vi "transfer table data.vi"(9 "transfer specification in":T1[](array[typedef]), 10 "data table source in":T3, 11 "data table sink in":T3) -> (1 "transfer specification out":T1[](array[typedef]), 2 "data table source out":T3, 3 "data table sink out":T3)   [LabVIEW 2013, in "tag bus.lvlib" / "data table.lvlib"]
doc: "Applies the data transfer between the source table and sink table, as defined by the transfer specification."
uses:
  data table.lvlib
  data table.ctl
  transfer specification.ctl
  tag/Data Type.ctl
  tag/tag descriptor.lvclass
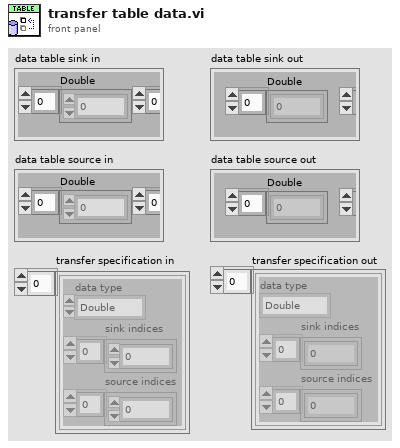
[diagram p1: front panel]
types:
  T1 = typedef "tag bus.lvlib/data table.lvlib/transfer specification.ctl" = cluster{"data type":T2, "sink indices":i32[], "source indices":i32[]}
  T2 = typedef "tag bus.lvlib/tag descriptor.lvclass/Data Type.ctl" = enum16{"Double", "Single", "I64", "I32", "I16", "I8", "U64", "U32", "U16", "U8", "Boolean", "String", "Array of Double", "Array of Single", "Array of I64", "Array of I32", "Array of I16", "Array of I8", "Array of U64", "Array of U32", "Array of U16", "Array of U8", "Array of Boolean", "Array of String"}
  T3 = typedef "tag bus.lvlib/data table.lvlib/data table.ctl" = cluster{"Double":dbl[], "Single":sgl[], "I64":i64[], "I32":i32[], "I16":i16[], "I8":i8[], "U64":u64[], "U32":u32[], "U16":u16[], "U8":u8[], "Boolean":bool[], "String":string[], "Array of Double":cluster{"DBL Array":dbl[]}[], "Array of Single":cluster{"SGL Array":sgl[]}[], "Array of I64":cluster{"I64 Array":i64[]}[], "Array of I32":cluster{"I32 Array":i32[]}[], "Array of I16":cluster{"I16 Array":i16[]}[], "Array of I8":cluster{"I8 Array":i8[]}[], "Array of U64":cluster{"U64 Array":u64[]}[], "Array of U32":cluster{"U32 Array":u32[]}[], "Array of U16":cluster{"U16 Array":u16[]}[], "Array of U8":cluster{"U8 Array":u8[]}[], "Array of Boolean":cluster{"Boolean Array":bool[]}[], "Array of String":cluster{"String Array":string[]}[]}
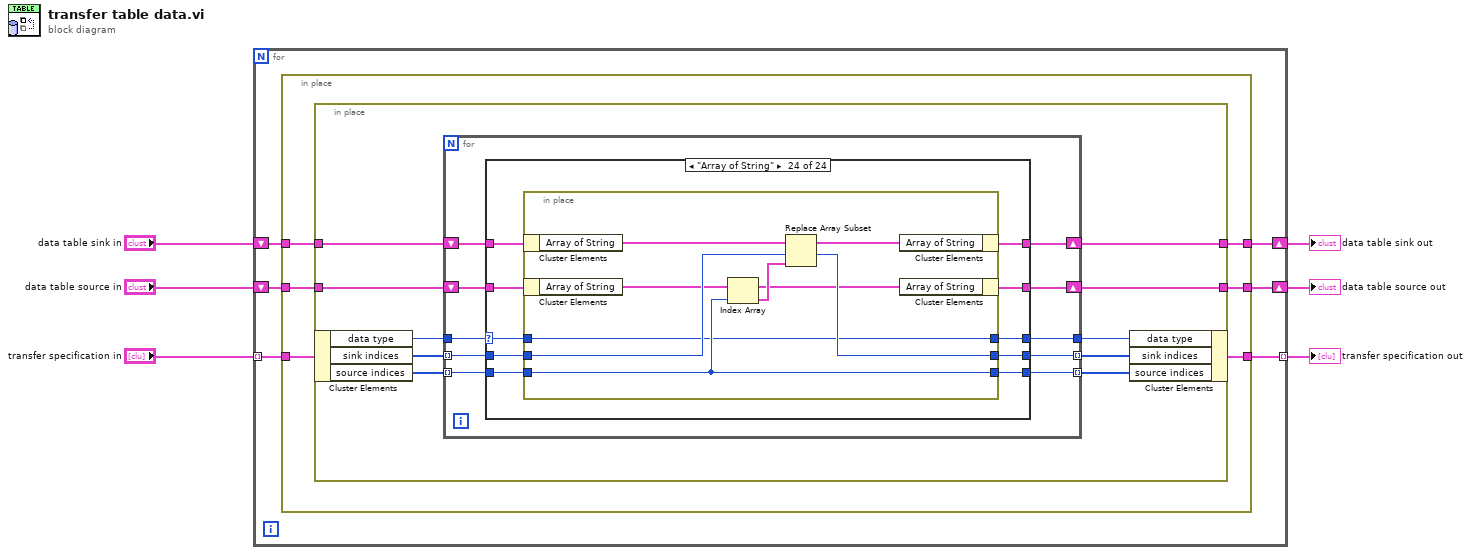
[diagram p0: block diagram]
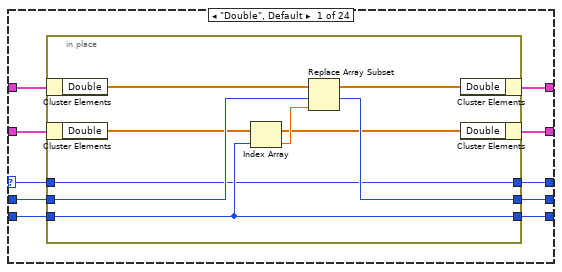
[diagram p2: hidden frame]
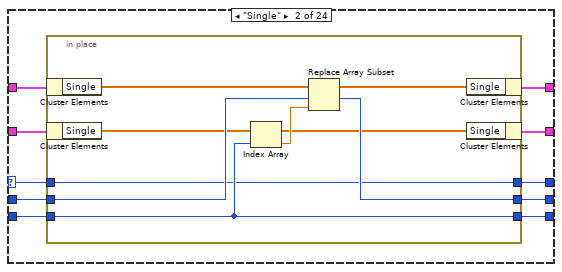
[diagram p3: hidden frame]
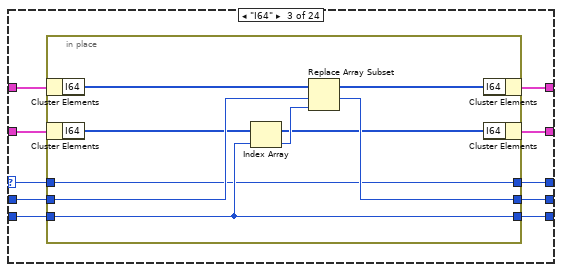
[diagram p4: hidden frame]
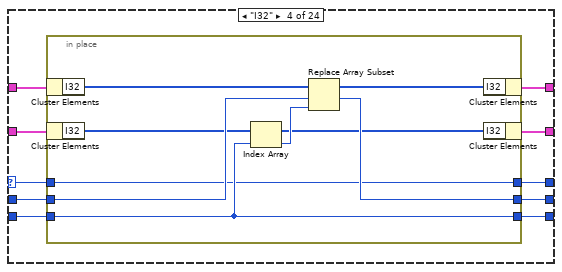
[diagram p5: hidden frame]
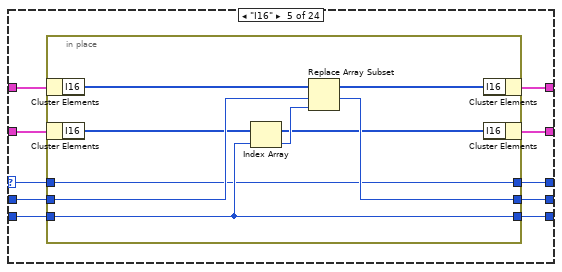
[diagram p6: hidden frame]
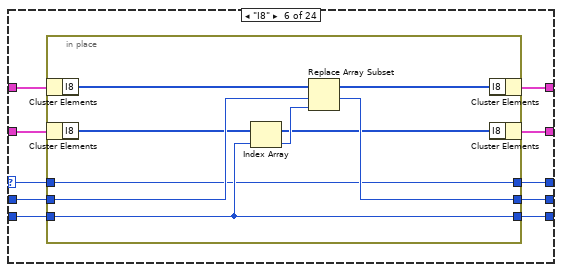
[diagram p7: hidden frame]
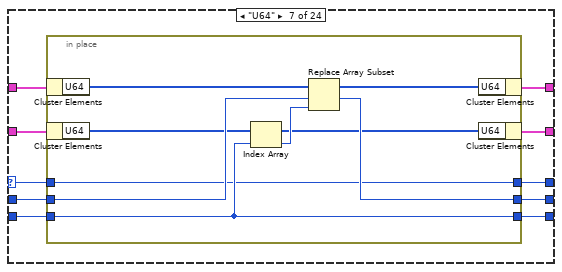
[diagram p8: hidden frame]
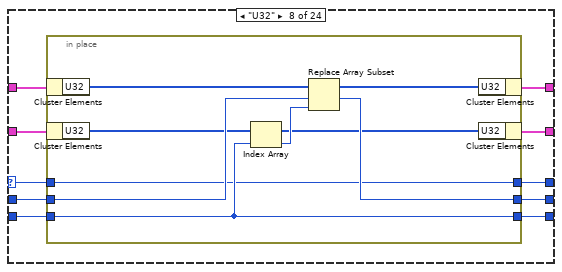
[diagram p9: hidden frame]
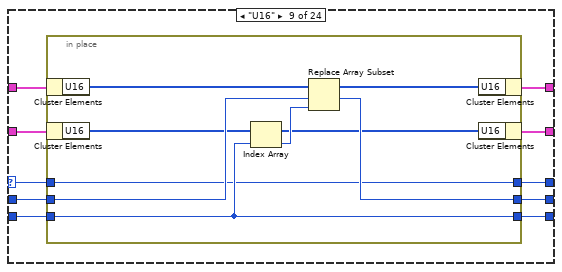
[diagram p10: hidden frame]
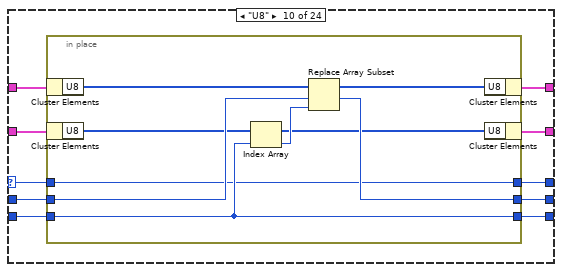
[diagram p11: hidden frame]
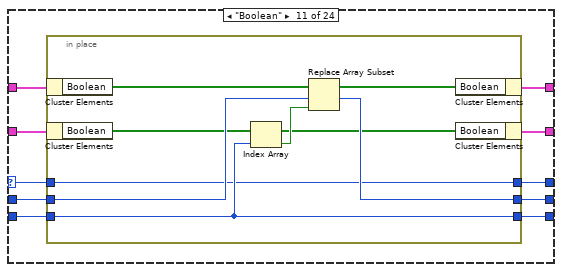
[diagram p12: hidden frame]
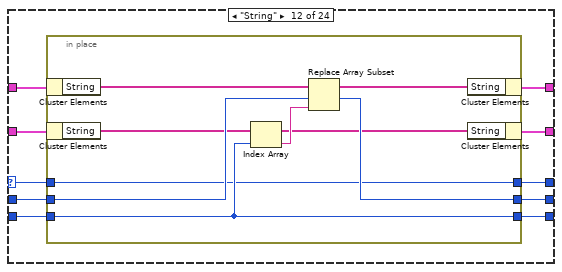
[diagram p13: hidden frame]
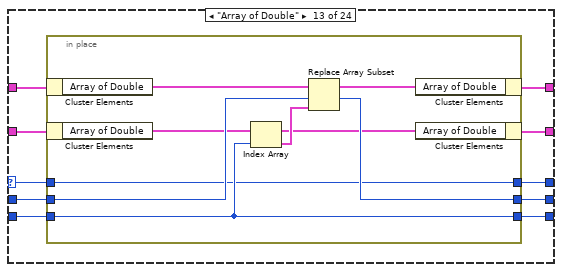
[diagram p14: hidden frame]
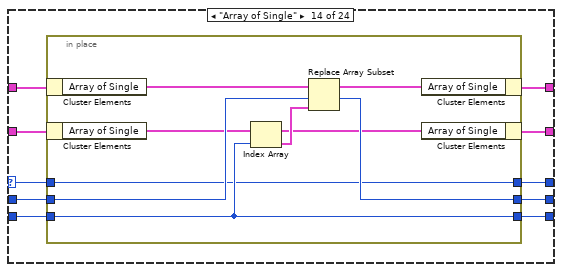
[diagram p15: hidden frame]
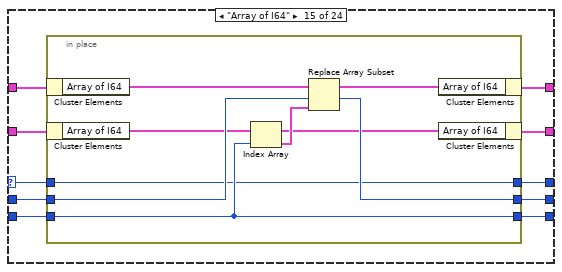
[diagram p16: hidden frame]
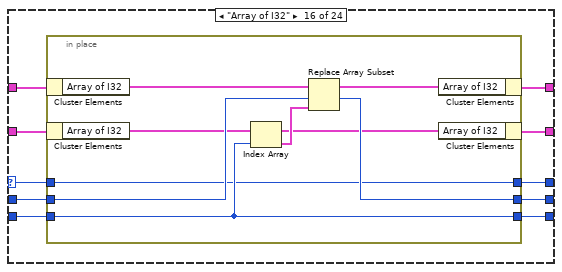
[diagram p17: hidden frame]
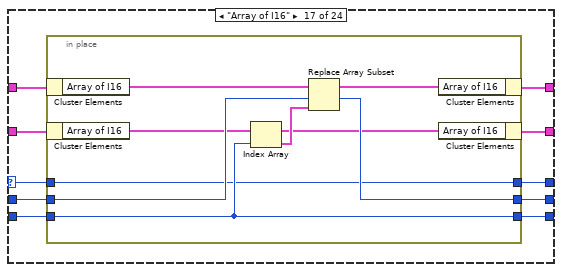
[diagram p18: hidden frame]
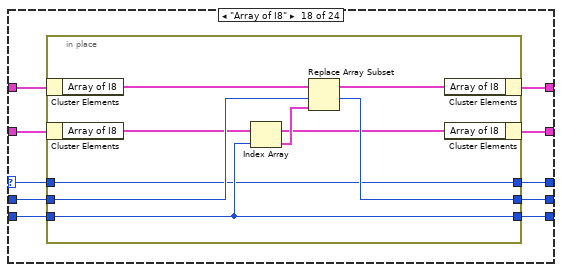
[diagram p19: hidden frame]
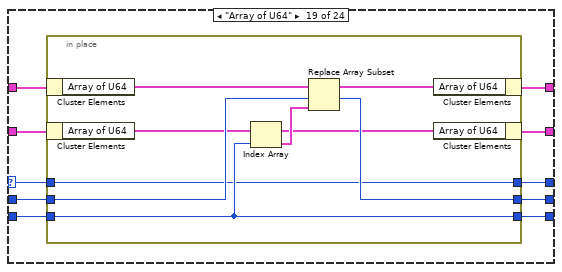
[diagram p20: hidden frame]
diagram:
  n1 = for {
    tunnel: "transfer specification in" -> [w8] mode=indexing
    shift-right: [w9] -> w2
    shift-left: "data table source in" -> [w10]
    shift-right: [w11] -> w3
    shift-left: "data table sink in" -> [w12]
    tunnel: [w7] -> w1 mode=indexing
    n2 = in-place {
      in-place-border: w12 -> [w18]
      in-place-border: [w17] -> w11
      in-place-border: w10 -> [w16]
      in-place-border: [w15] -> w9
      in-place-border: w8 -> [w14]
      in-place-border: [w13] -> w7
      n3 = in-place {
        in-place-border: w18 -> [w28]
        in-place-border: [w27] -> w17
        in-place-border: w16 -> [w26]
        in-place-border: [w25] -> w15
        n4 = in-place-cluster #1(w14) -> ("data type"=w24:T2, "sink indices"=w23:i32[], "source indices"=w22:i32[])
        n5 = for {
          shift-right: [w36] -> w27
          shift-left: w28 -> [w37]
          shift-right: [w35] -> w25
          shift-left: w26 -> [w34]
          tunnel: w24 -> [w38]
          tunnel: w23 -> [w33] mode=indexing
          tunnel: w22 -> [w32] mode=indexing
          tunnel: [w31] -> w21 mode=indexing
          tunnel: [w30] -> w20 mode=indexing
          tunnel: [w29] -> w19
          n6 = case shown="\"Array of String\"" w38 {
            selector: w38 -> [w40 w57 w74 w91 w108 w125 w142 w159 w176 w193 w210 w227 w244 w261 w278 w295 w312 w329 w346 w363 w380 w397 w414 w431]
            tunnel: w37 -> [w48 w65 w82 w99 w116 w133 w150 w167 w184 w201 w218 w235 w252 w269 w286 w303 w320 w337 w354 w371 w388 w405 w422 w439]
            tunnel: [w46 w63 w80 w97 w114 w131 w148 w165 w182 w199 w216 w233 w250 w267 w284 w301 w318 w335 w352 w369 w386 w403 w420 w437] -> w36
            tunnel: [w45 w62 w79 w96 w113 w130 w147 w164 w181 w198 w215 w232 w249 w266 w283 w300 w317 w334 w351 w368 w385 w402 w419 w436] -> w35
            tunnel: w34 -> [w47 w64 w81 w98 w115 w132 w149 w166 w183 w200 w217 w234 w251 w268 w285 w302 w319 w336 w353 w370 w387 w404 w421 w438]
            tunnel: w33 -> [w44 w61 w78 w95 w112 w129 w146 w163 w180 w197 w214 w231 w248 w265 w282 w299 w316 w333 w350 w367 w384 w401 w418 w435]
            tunnel: w32 -> [w43 w60 w77 w94 w111 w128 w145 w162 w179 w196 w213 w230 w247 w264 w281 w298 w315 w332 w349 w366 w383 w400 w417 w434]
            tunnel: [w42 w59 w76 w93 w110 w127 w144 w161 w178 w195 w212 w229 w246 w263 w280 w297 w314 w331 w348 w365 w382 w399 w416 w433] -> w31
            tunnel: [w41 w58 w75 w92 w109 w126 w143 w160 w177 w194 w211 w228 w245 w262 w279 w296 w313 w330 w347 w364 w381 w398 w415 w432] -> w30
            tunnel: [w39 w56 w73 w90 w107 w124 w141 w158 w175 w192 w209 w226 w243 w260 w277 w294 w311 w328 w345 w362 w379 w396 w413 w430] -> w29
            frame "Double", Default {
              n7 = in-place {
                in-place-border: w44 -> [w53]
                in-place-border: w43 -> [w52]
                in-place-border: [w53] -> w42
                in-place-border: [w52] -> w41
                in-place-border: w40 -> [w51]
                in-place-border: [w51] -> w39
                n8 = in-place-cluster #2(w48) -> ("Double"=w55:dbl[])
                n9 = in-place-cluster #3(w47) -> ("Double"=w49:dbl[])
                n10 = Index Array(array=w49, index=w52) -> (element=w50:dbl)
                n11 = Replace Array Subset(array=w55, new element=w50, index=w53) -> (w54:dbl[])
                n12 = in-place-cluster #2("Double"=w54) -> (w46:T3)
                n13 = in-place-cluster #3("Double"=w49) -> (w45:T3)
              }
            }
            frame "Single" {
              n14 = in-place {
                in-place-border: w61 -> [w70]
                in-place-border: w60 -> [w69]
                in-place-border: [w70] -> w59
                in-place-border: [w69] -> w58
                in-place-border: w57 -> [w68]
                in-place-border: [w68] -> w56
                n15 = in-place-cluster #4(w65) -> ("Single"=w72:sgl[])
                n16 = in-place-cluster #5(w64) -> ("Single"=w66:sgl[])
                n17 = Index Array(array=w66, index=w69) -> (element=w67:sgl)
                n18 = Replace Array Subset(array=w72, new element=w67, index=w70) -> (w71:sgl[])
                n19 = in-place-cluster #4("Single"=w71) -> (w63:T3)
                n20 = in-place-cluster #5("Single"=w66) -> (w62:T3)
              }
            }
            frame "I64" {
              n21 = in-place {
                in-place-border: w78 -> [w87]
                in-place-border: w77 -> [w86]
                in-place-border: [w87] -> w76
                in-place-border: [w86] -> w75
                in-place-border: w74 -> [w85]
                in-place-border: [w85] -> w73
                n22 = in-place-cluster #6(w82) -> ("I64"=w89:i64[])
                n23 = in-place-cluster #7(w81) -> ("I64"=w83:i64[])
                n24 = Index Array(array=w83, index=w86) -> (element=w84:i64)
                n25 = Replace Array Subset(array=w89, new element=w84, index=w87) -> (w88:i64[])
                n26 = in-place-cluster #6("I64"=w88) -> (w80:T3)
                n27 = in-place-cluster #7("I64"=w83) -> (w79:T3)
              }
            }
            frame "I32" {
              n28 = in-place {
                in-place-border: w95 -> [w104]
                in-place-border: w94 -> [w103]
                in-place-border: [w104] -> w93
                in-place-border: [w103] -> w92
                in-place-border: w91 -> [w102]
                in-place-border: [w102] -> w90
                n29 = in-place-cluster #8(w99) -> ("I32"=w106:i32[])
                n30 = in-place-cluster #9(w98) -> ("I32"=w100:i32[])
                n31 = Index Array(array=w100, index=w103) -> (element=w101:i32)
                n32 = Replace Array Subset(array=w106, new element=w101, index=w104) -> (w105:i32[])
                n33 = in-place-cluster #8("I32"=w105) -> (w97:T3)
                n34 = in-place-cluster #9("I32"=w100) -> (w96:T3)
              }
            }
            frame "I16" {
              n35 = in-place {
                in-place-border: w112 -> [w121]
                in-place-border: w111 -> [w120]
                in-place-border: [w121] -> w110
                in-place-border: [w120] -> w109
                in-place-border: w108 -> [w119]
                in-place-border: [w119] -> w107
                n36 = in-place-cluster #10(w116) -> ("I16"=w123:i16[])
                n37 = in-place-cluster #11(w115) -> ("I16"=w117:i16[])
                n38 = Index Array(array=w117, index=w120) -> (element=w118:i16)
                n39 = Replace Array Subset(array=w123, new element=w118, index=w121) -> (w122:i16[])
                n40 = in-place-cluster #10("I16"=w122) -> (w114:T3)
                n41 = in-place-cluster #11("I16"=w117) -> (w113:T3)
              }
            }
            frame "I8" {
              n42 = in-place {
                in-place-border: w129 -> [w138]
                in-place-border: w128 -> [w137]
                in-place-border: [w138] -> w127
                in-place-border: [w137] -> w126
                in-place-border: w125 -> [w136]
                in-place-border: [w136] -> w124
                n43 = in-place-cluster #12(w133) -> ("I8"=w140:i8[])
                n44 = in-place-cluster #13(w132) -> ("I8"=w134:i8[])
                n45 = Index Array(array=w134, index=w137) -> (element=w135:i8)
                n46 = Replace Array Subset(array=w140, new element=w135, index=w138) -> (w139:i8[])
                n47 = in-place-cluster #12("I8"=w139) -> (w131:T3)
                n48 = in-place-cluster #13("I8"=w134) -> (w130:T3)
              }
            }
            frame "U64" {
              n49 = in-place {
                in-place-border: w146 -> [w155]
                in-place-border: w145 -> [w154]
                in-place-border: [w155] -> w144
                in-place-border: [w154] -> w143
                in-place-border: w142 -> [w153]
                in-place-border: [w153] -> w141
                n50 = in-place-cluster #14(w150) -> ("U64"=w157:u64[])
                n51 = in-place-cluster #15(w149) -> ("U64"=w151:u64[])
                n52 = Index Array(array=w151, index=w154) -> (element=w152:u64)
                n53 = Replace Array Subset(array=w157, new element=w152, index=w155) -> (w156:u64[])
                n54 = in-place-cluster #14("U64"=w156) -> (w148:T3)
                n55 = in-place-cluster #15("U64"=w151) -> (w147:T3)
              }
            }
            frame "U32" {
              n56 = in-place {
                in-place-border: w163 -> [w172]
                in-place-border: w162 -> [w171]
                in-place-border: [w172] -> w161
                in-place-border: [w171] -> w160
                in-place-border: w159 -> [w170]
                in-place-border: [w170] -> w158
                n57 = in-place-cluster #16(w167) -> ("U32"=w174:u32[])
                n58 = in-place-cluster #17(w166) -> ("U32"=w168:u32[])
                n59 = Index Array(array=w168, index=w171) -> (element=w169:u32)
                n60 = Replace Array Subset(array=w174, new element=w169, index=w172) -> (w173:u32[])
                n61 = in-place-cluster #16("U32"=w173) -> (w165:T3)
                n62 = in-place-cluster #17("U32"=w168) -> (w164:T3)
              }
            }
            frame "U16" {
              n63 = in-place {
                in-place-border: w180 -> [w189]
                in-place-border: w179 -> [w188]
                in-place-border: [w189] -> w178
                in-place-border: [w188] -> w177
                in-place-border: w176 -> [w187]
                in-place-border: [w187] -> w175
                n64 = in-place-cluster #18(w184) -> ("U16"=w191:u16[])
                n65 = in-place-cluster #19(w183) -> ("U16"=w185:u16[])
                n66 = Index Array(array=w185, index=w188) -> (element=w186:u16)
                n67 = Replace Array Subset(array=w191, new element=w186, index=w189) -> (w190:u16[])
                n68 = in-place-cluster #18("U16"=w190) -> (w182:T3)
                n69 = in-place-cluster #19("U16"=w185) -> (w181:T3)
              }
            }
            frame "U8" {
              n70 = in-place {
                in-place-border: w197 -> [w206]
                in-place-border: w196 -> [w205]
                in-place-border: [w206] -> w195
                in-place-border: [w205] -> w194
                in-place-border: w193 -> [w204]
                in-place-border: [w204] -> w192
                n71 = in-place-cluster #20(w201) -> ("U8"=w208:u8[])
                n72 = in-place-cluster #21(w200) -> ("U8"=w202:u8[])
                n73 = Index Array(array=w202, index=w205) -> (element=w203:u8)
                n74 = Replace Array Subset(array=w208, new element=w203, index=w206) -> (w207:u8[])
                n75 = in-place-cluster #20("U8"=w207) -> (w199:T3)
                n76 = in-place-cluster #21("U8"=w202) -> (w198:T3)
              }
            }
            frame "Boolean" {
              n77 = in-place {
                in-place-border: w214 -> [w223]
                in-place-border: w213 -> [w222]
                in-place-border: [w223] -> w212
                in-place-border: [w222] -> w211
                in-place-border: w210 -> [w221]
                in-place-border: [w221] -> w209
                n78 = in-place-cluster #22(w218) -> ("Boolean"=w225:bool[])
                n79 = in-place-cluster #23(w217) -> ("Boolean"=w219:bool[])
                n80 = Index Array(array=w219, index=w222) -> (element=w220:bool)
                n81 = Replace Array Subset(array=w225, new element=w220, index=w223) -> (w224:bool[])
                n82 = in-place-cluster #22("Boolean"=w224) -> (w216:T3)
                n83 = in-place-cluster #23("Boolean"=w219) -> (w215:T3)
              }
            }
            frame "String" {
              n84 = in-place {
                in-place-border: w231 -> [w240]
                in-place-border: w230 -> [w239]
                in-place-border: [w240] -> w229
                in-place-border: [w239] -> w228
                in-place-border: w227 -> [w238]
                in-place-border: [w238] -> w226
                n85 = in-place-cluster #24(w235) -> ("String"=w242:string[])
                n86 = in-place-cluster #25(w234) -> ("String"=w236:string[])
                n87 = Index Array(array=w236, index=w239) -> (element=w237:string)
                n88 = Replace Array Subset(array=w242, new element=w237, index=w240) -> (w241:string[])
                n89 = in-place-cluster #24("String"=w241) -> (w233:T3)
                n90 = in-place-cluster #25("String"=w236) -> (w232:T3)
              }
            }
            frame "Array of Double" {
              n91 = in-place {
                in-place-border: w248 -> [w257]
                in-place-border: w247 -> [w256]
                in-place-border: [w257] -> w246
                in-place-border: [w256] -> w245
                in-place-border: w244 -> [w255]
                in-place-border: [w255] -> w243
                n92 = in-place-cluster #26(w252) -> ("Array of Double"=w259:cluster{"DBL Array":dbl[]}[])
                n93 = in-place-cluster #27(w251) -> ("Array of Double"=w253:cluster{"DBL Array":dbl[]}[])
                n94 = Index Array(array=w253, index=w256) -> (element=w254:cluster{"DBL Array":dbl[]})
                n95 = Replace Array Subset(array=w259, new element=w254, index=w257) -> (w258:cluster{"DBL Array":dbl[]}[])
                n96 = in-place-cluster #26("Array of Double"=w258) -> (w250:T3)
                n97 = in-place-cluster #27("Array of Double"=w253) -> (w249:T3)
              }
            }
            frame "Array of Single" {
              n98 = in-place {
                in-place-border: w265 -> [w274]
                in-place-border: w264 -> [w273]
                in-place-border: [w274] -> w263
                in-place-border: [w273] -> w262
                in-place-border: w261 -> [w272]
                in-place-border: [w272] -> w260
                n99 = in-place-cluster #28(w269) -> ("Array of Single"=w276:cluster{"SGL Array":sgl[]}[])
                n100 = in-place-cluster #29(w268) -> ("Array of Single"=w270:cluster{"SGL Array":sgl[]}[])
                n101 = Index Array(array=w270, index=w273) -> (element=w271:cluster{"SGL Array":sgl[]})
                n102 = Replace Array Subset(array=w276, new element=w271, index=w274) -> (w275:cluster{"SGL Array":sgl[]}[])
                n103 = in-place-cluster #28("Array of Single"=w275) -> (w267:T3)
                n104 = in-place-cluster #29("Array of Single"=w270) -> (w266:T3)
              }
            }
            frame "Array of I64" {
              n105 = in-place {
                in-place-border: w282 -> [w291]
                in-place-border: w281 -> [w290]
                in-place-border: [w291] -> w280
                in-place-border: [w290] -> w279
                in-place-border: w278 -> [w289]
                in-place-border: [w289] -> w277
                n106 = in-place-cluster #30(w286) -> ("Array of I64"=w293:cluster{"I64 Array":i64[]}[])
                n107 = in-place-cluster #31(w285) -> ("Array of I64"=w287:cluster{"I64 Array":i64[]}[])
                n108 = Index Array(array=w287, index=w290) -> (element=w288:cluster{"I64 Array":i64[]})
                n109 = Replace Array Subset(array=w293, new element=w288, index=w291) -> (w292:cluster{"I64 Array":i64[]}[])
                n110 = in-place-cluster #30("Array of I64"=w292) -> (w284:T3)
                n111 = in-place-cluster #31("Array of I64"=w287) -> (w283:T3)
              }
            }
            frame "Array of I32" {
              n112 = in-place {
                in-place-border: w299 -> [w308]
                in-place-border: w298 -> [w307]
                in-place-border: [w308] -> w297
                in-place-border: [w307] -> w296
                in-place-border: w295 -> [w306]
                in-place-border: [w306] -> w294
                n113 = in-place-cluster #32(w303) -> ("Array of I32"=w310:cluster{"I32 Array":i32[]}[])
                n114 = in-place-cluster #33(w302) -> ("Array of I32"=w304:cluster{"I32 Array":i32[]}[])
                n115 = Index Array(array=w304, index=w307) -> (element=w305:cluster{"I32 Array":i32[]})
                n116 = Replace Array Subset(array=w310, new element=w305, index=w308) -> (w309:cluster{"I32 Array":i32[]}[])
                n117 = in-place-cluster #32("Array of I32"=w309) -> (w301:T3)
                n118 = in-place-cluster #33("Array of I32"=w304) -> (w300:T3)
              }
            }
            frame "Array of I16" {
              n119 = in-place {
                in-place-border: w316 -> [w325]
                in-place-border: w315 -> [w324]
                in-place-border: [w325] -> w314
                in-place-border: [w324] -> w313
                in-place-border: w312 -> [w323]
                in-place-border: [w323] -> w311
                n120 = in-place-cluster #34(w320) -> ("Array of I16"=w327:cluster{"I16 Array":i16[]}[])
                n121 = in-place-cluster #35(w319) -> ("Array of I16"=w321:cluster{"I16 Array":i16[]}[])
                n122 = Index Array(array=w321, index=w324) -> (element=w322:cluster{"I16 Array":i16[]})
                n123 = Replace Array Subset(array=w327, new element=w322, index=w325) -> (w326:cluster{"I16 Array":i16[]}[])
                n124 = in-place-cluster #34("Array of I16"=w326) -> (w318:T3)
                n125 = in-place-cluster #35("Array of I16"=w321) -> (w317:T3)
              }
            }
            frame "Array of I8" {
              n126 = in-place {
                in-place-border: w333 -> [w342]
                in-place-border: w332 -> [w341]
                in-place-border: [w342] -> w331
                in-place-border: [w341] -> w330
                in-place-border: w329 -> [w340]
                in-place-border: [w340] -> w328
                n127 = in-place-cluster #36(w337) -> ("Array of I8"=w344:cluster{"I8 Array":i8[]}[])
                n128 = in-place-cluster #37(w336) -> ("Array of I8"=w338:cluster{"I8 Array":i8[]}[])
                n129 = Index Array(array=w338, index=w341) -> (element=w339:cluster{"I8 Array":i8[]})
                n130 = Replace Array Subset(array=w344, new element=w339, index=w342) -> (w343:cluster{"I8 Array":i8[]}[])
                n131 = in-place-cluster #36("Array of I8"=w343) -> (w335:T3)
                n132 = in-place-cluster #37("Array of I8"=w338) -> (w334:T3)
              }
            }
            frame "Array of U64" {
              n133 = in-place {
                in-place-border: w350 -> [w359]
                in-place-border: w349 -> [w358]
                in-place-border: [w359] -> w348
                in-place-border: [w358] -> w347
                in-place-border: w346 -> [w357]
                in-place-border: [w357] -> w345
                n134 = in-place-cluster #38(w354) -> ("Array of U64"=w361:cluster{"U64 Array":u64[]}[])
                n135 = in-place-cluster #39(w353) -> ("Array of U64"=w355:cluster{"U64 Array":u64[]}[])
                n136 = Index Array(array=w355, index=w358) -> (element=w356:cluster{"U64 Array":u64[]})
                n137 = Replace Array Subset(array=w361, new element=w356, index=w359) -> (w360:cluster{"U64 Array":u64[]}[])
                n138 = in-place-cluster #38("Array of U64"=w360) -> (w352:T3)
                n139 = in-place-cluster #39("Array of U64"=w355) -> (w351:T3)
              }
            }
            frame "Array of U32" {
              n140 = in-place {
                in-place-border: w367 -> [w376]
                in-place-border: w366 -> [w375]
                in-place-border: [w376] -> w365
                in-place-border: [w375] -> w364
                in-place-border: w363 -> [w374]
                in-place-border: [w374] -> w362
                n141 = in-place-cluster #40(w371) -> ("Array of U32"=w378:cluster{"U32 Array":u32[]}[])
                n142 = in-place-cluster #41(w370) -> ("Array of U32"=w372:cluster{"U32 Array":u32[]}[])
                n143 = Index Array(array=w372, index=w375) -> (element=w373:cluster{"U32 Array":u32[]})
                n144 = Replace Array Subset(array=w378, new element=w373, index=w376) -> (w377:cluster{"U32 Array":u32[]}[])
                n145 = in-place-cluster #40("Array of U32"=w377) -> (w369:T3)
                n146 = in-place-cluster #41("Array of U32"=w372) -> (w368:T3)
              }
            }
            frame "Array of U16" {
              n147 = in-place {
                in-place-border: w384 -> [w393]
                in-place-border: w383 -> [w392]
                in-place-border: [w393] -> w382
                in-place-border: [w392] -> w381
                in-place-border: w380 -> [w391]
                in-place-border: [w391] -> w379
                n148 = in-place-cluster #42(w388) -> ("Array of U16"=w395:cluster{"U16 Array":u16[]}[])
                n149 = in-place-cluster #43(w387) -> ("Array of U16"=w389:cluster{"U16 Array":u16[]}[])
                n150 = Index Array(array=w389, index=w392) -> (element=w390:cluster{"U16 Array":u16[]})
                n151 = Replace Array Subset(array=w395, new element=w390, index=w393) -> (w394:cluster{"U16 Array":u16[]}[])
                n152 = in-place-cluster #42("Array of U16"=w394) -> (w386:T3)
                n153 = in-place-cluster #43("Array of U16"=w389) -> (w385:T3)
              }
            }
            frame "Array of U8" {
              n154 = in-place {
                in-place-border: w401 -> [w410]
                in-place-border: w400 -> [w409]
                in-place-border: [w410] -> w399
                in-place-border: [w409] -> w398
                in-place-border: w397 -> [w408]
                in-place-border: [w408] -> w396
                n155 = in-place-cluster #44(w405) -> ("Array of U8"=w412:cluster{"U8 Array":u8[]}[])
                n156 = in-place-cluster #45(w404) -> ("Array of U8"=w406:cluster{"U8 Array":u8[]}[])
                n157 = Index Array(array=w406, index=w409) -> (element=w407:cluster{"U8 Array":u8[]})
                n158 = Replace Array Subset(array=w412, new element=w407, index=w410) -> (w411:cluster{"U8 Array":u8[]}[])
                n159 = in-place-cluster #44("Array of U8"=w411) -> (w403:T3)
                n160 = in-place-cluster #45("Array of U8"=w406) -> (w402:T3)
              }
            }
            frame "Array of Boolean" {
              n161 = in-place {
                in-place-border: w418 -> [w427]
                in-place-border: w417 -> [w426]
                in-place-border: [w427] -> w416
                in-place-border: [w426] -> w415
                in-place-border: w414 -> [w425]
                in-place-border: [w425] -> w413
                n162 = in-place-cluster #46(w422) -> ("Array of Boolean"=w429:cluster{"Boolean Array":bool[]}[])
                n163 = in-place-cluster #47(w421) -> ("Array of Boolean"=w423:cluster{"Boolean Array":bool[]}[])
                n164 = Index Array(array=w423, index=w426) -> (element=w424:cluster{"Boolean Array":bool[]})
                n165 = Replace Array Subset(array=w429, new element=w424, index=w427) -> (w428:cluster{"Boolean Array":bool[]}[])
                n166 = in-place-cluster #46("Array of Boolean"=w428) -> (w420:T3)
                n167 = in-place-cluster #47("Array of Boolean"=w423) -> (w419:T3)
              }
            }
            frame "Array of String" {
              n168 = in-place {
                in-place-border: w435 -> [w444]
                in-place-border: w434 -> [w443]
                in-place-border: [w444] -> w433
                in-place-border: [w443] -> w432
                in-place-border: w431 -> [w442]
                in-place-border: [w442] -> w430
                n169 = in-place-cluster #48(w439) -> ("Array of String"=w446:cluster{"String Array":string[]}[])
                n170 = in-place-cluster #49(w438) -> ("Array of String"=w440:cluster{"String Array":string[]}[])
                n171 = Index Array(array=w440, index=w443) -> (element=w441:cluster{"String Array":string[]})
                n172 = Replace Array Subset(array=w446, new element=w441, index=w444) -> (w445:cluster{"String Array":string[]}[])
                n173 = in-place-cluster #48("Array of String"=w445) -> (w437:T3)
                n174 = in-place-cluster #49("Array of String"=w440) -> (w436:T3)
              }
            }
          }
        }
        n175 = in-place-cluster #1("data type"=w19, "sink indices"=w21, "source indices"=w20) -> (w13:T1)
      }
    }
  }
  "data table sink out" <- w3
  "data table source out" <- w2
  "transfer specification out" <- w1
